vi "7170string to array.vi"(4 "Array in":string[](array[string])) -> (1 "Array out":dbl[](array[numeric]))   [LabVIEW 2014]
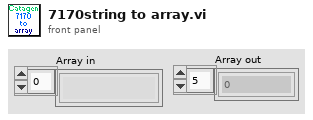
[diagram p1: front panel]
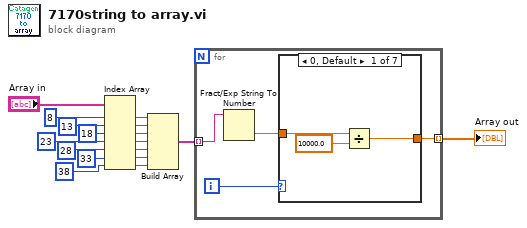
[diagram p0: block diagram]
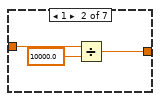
[diagram p2: hidden frame]
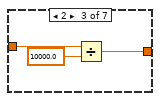
[diagram p3: hidden frame]
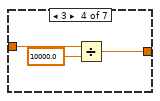
[diagram p4: hidden frame]
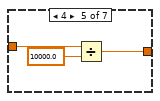
[diagram p5: hidden frame]
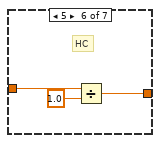
[diagram p6: hidden frame]
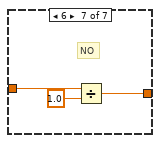
[diagram p7: hidden frame]
diagram:
  n1 = Index Array(array="Array in", index #1=8 ("index"), index #2=13 ("index"), index #3=18 ("index"), index #4=23 ("index"), index #5=28 ("index"), index #6=33 ("index"), index #7=38 ("index")) -> (element #1=w9:string, element #2=w8:string, element #3=w7:string, element #4=w6:string, element #5=w5:string, element #6=w4:string, element #7=w3:string)
  n2 = Build Array(w9, w8, w7, w6, w5, w4, w3) -> (w2:string[])
  n3 = for {
    tunnel: w2 -> [w20] mode=indexing
    tunnel: [w18] -> w1 mode=indexing
    i -> [w21]
    n4 = Fract/Exp String To Number(string=w20) -> (number=w19:dbl)  [unwired: 3 in, 1 out]
    n5 = case shown="0, Default" w21 {
      tunnel: w19 -> [w24 w25 w28 w31 w34 w37 w40]
      tunnel: [w22 w26 w29 w32 w35 w38 w41] -> w18
      frame 0, Default {
        n6 = Divide(x=w24, y=10000.0) -> (x/y=w22:dbl)
      }
      frame 1 {
        n7 = Divide(x=w25, y=10000.0) -> (x/y=w26:dbl)
      }
      frame 2 {
        n8 = Divide(x=w28, y=10000.0) -> (x/y=w29:dbl)
      }
      frame 3 {
        n9 = Divide(x=w31, y=10000.0) -> (x/y=w32:dbl)
      }
      frame 4 {
        n10 = Divide(x=w34, y=10000.0) -> (x/y=w35:dbl)
      }
      frame 5 {
        # "HC"
        n11 = Divide(x=w37, y=1.0) -> (x/y=w38:dbl)
      }
      frame 6 {
        # "NO"
        n12 = Divide(x=w40, y=1.0) -> (x/y=w41:dbl)
      }
    }
  }
  "Array out" <- w1
